vi "Send Action To Server.vi"(7 "moves":cluster{i32, i32, i32}, 8 "error in (no error)":errorcluster, 9 "role":string, 10 "match_id":string, 11 "Refnum in":refnum<k35>) -> (0 "error out":errorcluster, 2 "String out":string, 3 "Refnum out":refnum<k35>)   [LabVIEW 2025]
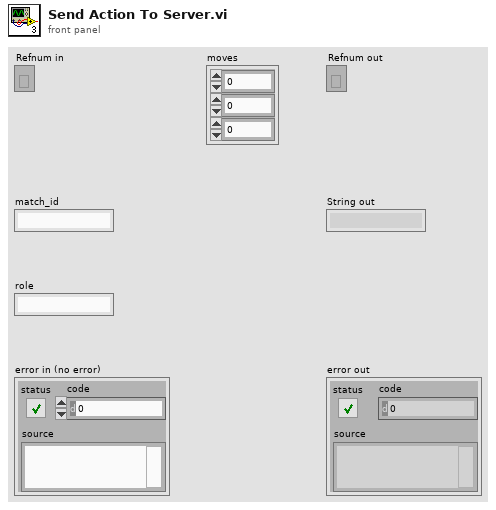
[diagram p1: front panel]
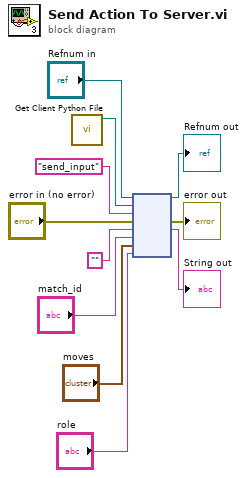
[diagram p0: block diagram]
diagram:
  n1 = call "Get Client Python File.vi"() -> ("appended path"=w5:path)  [unwired: 11 in]
  n2 = node("Refnum in", w5, "send_input" ("function name"), "error in (no error)", "", "match_id", "moves", "role") -> (→"Refnum out":refnum<k35>, →"error out":errorcluster, →"String out":string)  [unwired: 3 in, 2 out]
